vi "Initialize Plugin.vi"(8 "error in":errorcluster) -> (0 "error out":errorcluster, 2 "Called From Framework? Yes (T) No (F)":bool, 3 "Event Registration Refnum":refnum<event-registration>)   [LabVIEW 2011, in "Generic Plugin.lvclass"]
uses:
  Plugin Template/Generic Plugin.lvclass
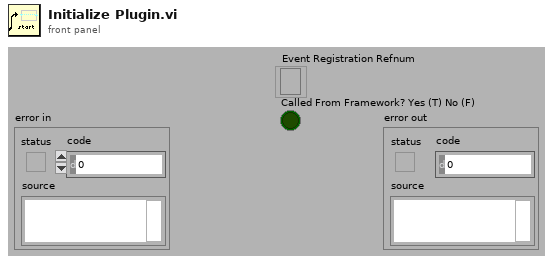
[diagram p1: front panel]
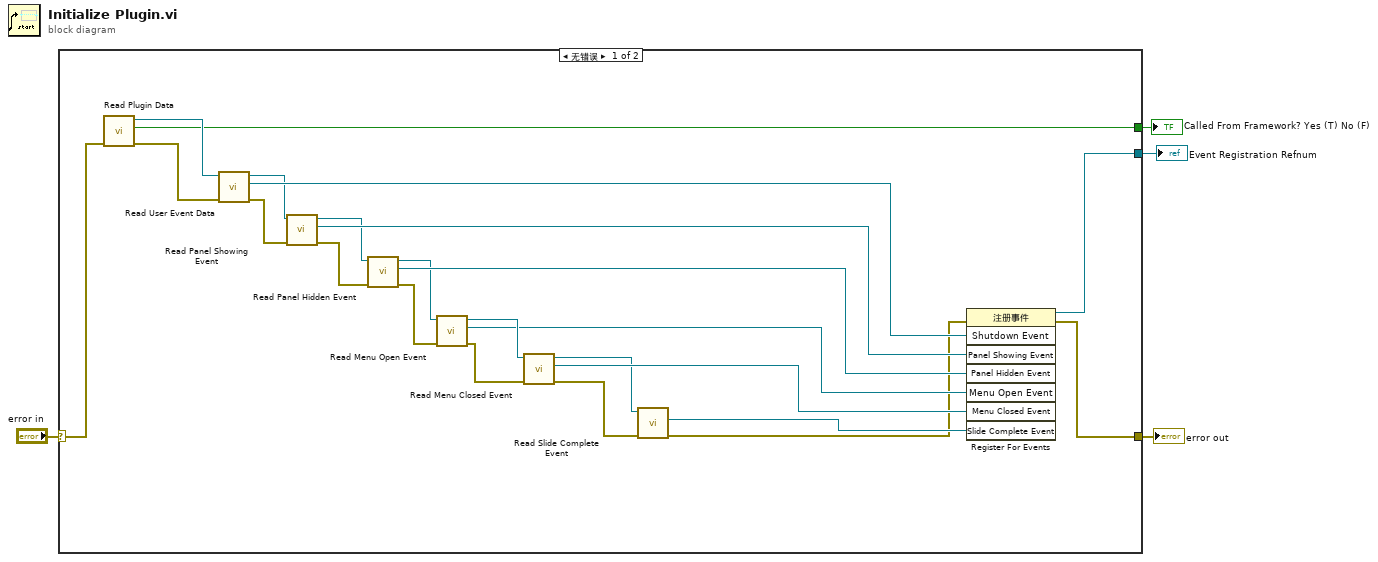
[diagram p0: block diagram]
diagram:
  n1 = case shown="无错误" "error in" {
    selector: "error in" -> [w23 w28]
    tunnel: [w27 w28] -> w4
    tunnel: [w7 _] -> w2
    tunnel: [w5 _] -> w1
    frame No Error {
      n2 = call "Read Plugin Data.vi"("error in (no error)"=w23) -> ("error out"=w26:errorcluster, "Queue Exists? Yes (T) No (F)"=w5:bool, "Plugin Data"=w24:refnum<class "Generic Plugin.lvclass">)  [unwired: 8 in]
      n3 = call "Read User Event Data.vi"("error in (no error)"=w26, "Generic Plugin in"=w24) -> ("error out"=w21:errorcluster, "Shutdown Event"=w25:refnum<user-event>, "Generic Plugin out"=w22:refnum<class "Generic Plugin.lvclass">)  [unwired: 7 in]
      n4 = call "Read Panel Showing Event.vi"("error in (no error)"=w21, "Generic Plugin in"=w22) -> ("error out"=w17:errorcluster, "Panel Showing Event"=w20:refnum<user-event>, "Generic Plugin out"=w18:refnum<class "Generic Plugin.lvclass">)  [unwired: 7 in]
      n5 = call "Read Panel Hidden Event.vi"("error in (no error)"=w17, "Generic Plugin in"=w18) -> ("error out"=w11:errorcluster, "Panel Hidden Event"=w19:refnum<user-event>, "Generic Plugin out"=w16:refnum<class "Generic Plugin.lvclass">)  [unwired: 7 in]
      n6 = call "Read Menu Open Event.vi"("error in (no error)"=w11, "Generic Plugin in"=w16) -> ("error out"=w12:errorcluster, "Menu Open Event"=w14:refnum<user-event>, "Generic Plugin out"=w15:refnum<class "Generic Plugin.lvclass">)  [unwired: 7 in]
      n7 = call "Read Menu Closed Event.vi"("error in (no error)"=w12, "Generic Plugin in"=w15) -> ("error out"=w9:errorcluster, "Menu Closed Event"=w13:refnum<user-event>, "Generic Plugin out"=w6:refnum<class "Generic Plugin.lvclass">)  [unwired: 7 in]
      n8 = call "Read Slide Complete Event.vi"("error in (no error)"=w9, "Generic Plugin in"=w6) -> ("error out"=w8:errorcluster, "Slide Complete Event"=w10:refnum<user-event>)  [unwired: 7 in, 1 out]
      n9 = register-events(error in=w8, w25, w20, w19, w14, w13, w10) -> (reference out=w7:refnum<event-registration>, error out=w27:errorcluster)  [unwired: 1 in]
    }
    frame Error {
    }
  }
  "error out" <- w4
  "Event Registration Refnum" <- w2
  "Called From Framework? Yes (T) No (F)" <- w1
